vi "Main - Auto Detect Modules.vi"(8 "error in (no error)":errorcluster, 11 "Node Ptr":u64 format="%.0x") -> (0 "error out":errorcluster)   [LabVIEW 2016, in "Scan Engine Custom Device.lvlib"]
uses:
  Scan Engine Custom Device.lvlib
  <vilib>/NI Veristand/Custom Device API/Custom Device Channel.ctl
  <vilib>/NI Veristand/Custom Device API/Custom Device Channel Type.ctl
  Modules.lvlibp/RSI Module/Slot Settings.ctl
  Modules.lvlibp/RSI Module/Module Models.ctl
  Type Defs/Host - FPGAScanInterfaceMode.ctl
  Globals/String Constants.vi
  Globals/Scan Engine GUIDs.vi
  Globals/Property Strings.vi
  Modules.lvlibp/RSI Module/Class Property Strings.vi
  Modules.lvlibp/RSI Module/RSI Module.lvclass
  Modules.lvlibp/RemIO Module/RemIO Module.lvclass
  <vilib>/NI Veristand/Custom Device API/Custom Device API.lvlib
  Modules.lvlibp
  <resource>/objmgr/ni.var.rc
panel:
  in  "Tag":string
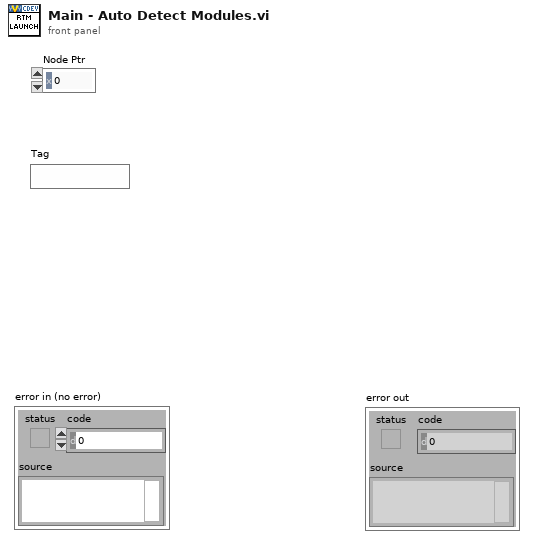
[diagram p1: front panel]
types:
  T1 = typedef "Custom Device API.lvlib/Custom Device Channel Type.ctl" = enum16{"Input", "Output"}
  T2 = typedef "Modules.lvlibp/RSI Module.lvclass/Slot Settings.ctl" = cluster{"Slot":u32, "EtherCAT?":bool}
  T3 = typedef "Modules.lvlibp/RSI Module.lvclass/Module Models.ctl" = enum16{"Empty", "NI 9201", "NI 9203", "NI 9205", "NI 9206", "NI 9207", "NI 9208", "NI 9211", "NI 9212", "NI 9213", "NI 9214", "NI 9215", "NI 9217", "NI 9219", "NI 9220", "NI 9221", "NI 9222", "NI 9223", "NI 9225", "NI 9227", "NI 9229", "NI 9233", "NI 9234", "NI 9235", "NI 9236", "NI 9237", "NI 9239", "NI 9242", "NI 9244", "NI 9263", "NI 9264", "NI 9265", "NI 9269", "NI 9375", "NI 9401", "NI 9402", "NI 9403", "NI 9411", "NI 9421", "NI 9422", "NI 9423", "NI 9425", "NI 9426", "NI 9435", "NI 9437", "NI 9472", "NI 9474", "NI 9475", "NI 9476", "NI 9477", "NI 9478", "NI 9481", "NI 9482", "NI 9485"}
  T4 = typedef "Scan Engine Custom Device.lvlib/Host - FPGAScanInterfaceMode.ctl" = enum16{"Use Current", "FPGA", "Scan Mode"}
  T5 = typedef "Custom Device API.lvlib/Custom Device Item Ref.ctl" = u64
  T6 = typedef "Custom Device API.lvlib/Custom Device Item Info.ctl" = cluster{"Name":string, "Is Channel":bool, "GUID":string, "Is Waveform":bool}
  T7 = typedef "Scan Engine Custom Device.lvlib/Host - HW Config.ctl" = cluster{"Local Chassis":T8, "Masters":T10[]}
  T8 = typedef "Scan Engine Custom Device.lvlib/Host - Local Chassis.ctl" = cluster{"Modules":T9[]}
  T9 = typedef "Scan Engine Custom Device.lvlib/Host - Module.ctl" = cluster{"IOV Ref":refnum<k21>, "Slot":u32, "Model":u32}
  T10 = typedef "Scan Engine Custom Device.lvlib/Host - Master.ctl" = cluster{"IOV Ref":refnum<k21>, "Name":string, "Master ID":u32, "Slaves":T11[]}
  T11 = typedef "Scan Engine Custom Device.lvlib/Host - Slave.ctl" = cluster{"IOV Ref":refnum<k21>, "Name":string, "Position Address":u16, "Bitfile Signature":u8[], "Modules":T9[], "ECAT Variablenobjekt":refnum<k21>[]}
  T12 = typedef "Custom Device API.lvlib/Custom Device Channel.ctl" = cluster{"Type":T1, "Units":string, "Default Value":dbl, "Faultable":bool, "Scalable":bool}
  T13 = typedef "Scan Engine Custom Device.lvlib/ECAT Channel Data Type.ctl" = enum16{"Boolean", "Fixed Point", "Int8", "Int16", "Int32", "Int64", "U32 Bit Field", "UInt8", "UInt16", "UInt32", "UInt64", "Other", "DBL"}
  T14 = typedef "Modules.lvlibp/Custom Device API.lvlib/Custom Device Item Ref.ctl" = u64
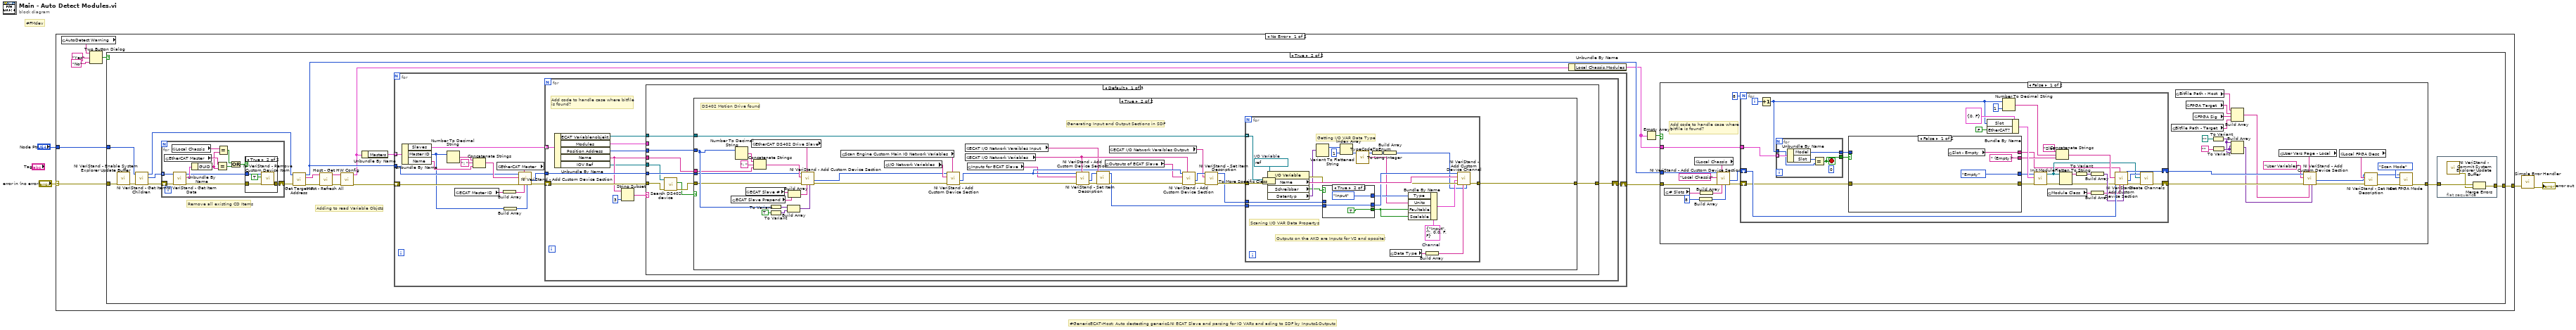
[diagram p0: block diagram]
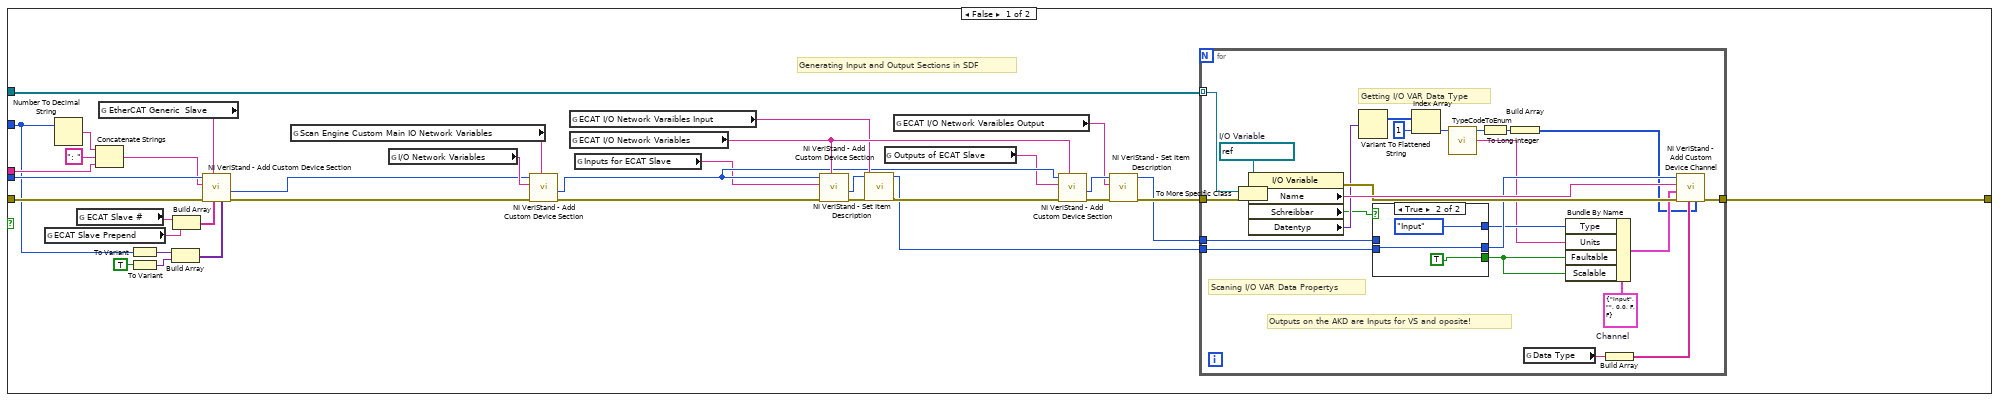
[diagram p3: hidden frame]
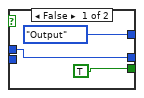
[diagram p4: hidden frame]
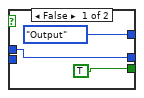
[diagram p5: hidden frame]
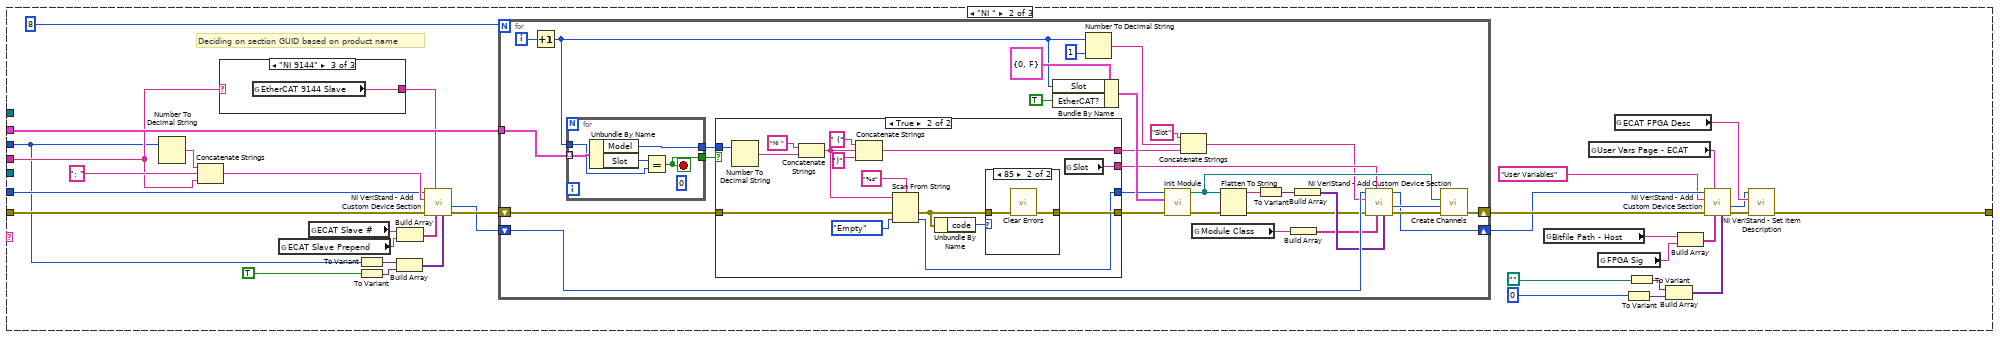
[diagram p6: hidden frame]
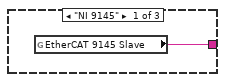
[diagram p7: hidden frame]
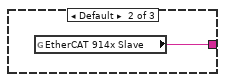
[diagram p8: hidden frame]
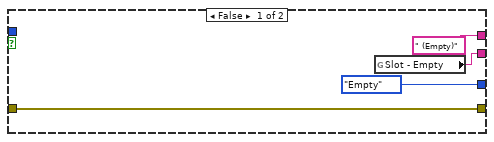
[diagram p9: hidden frame]
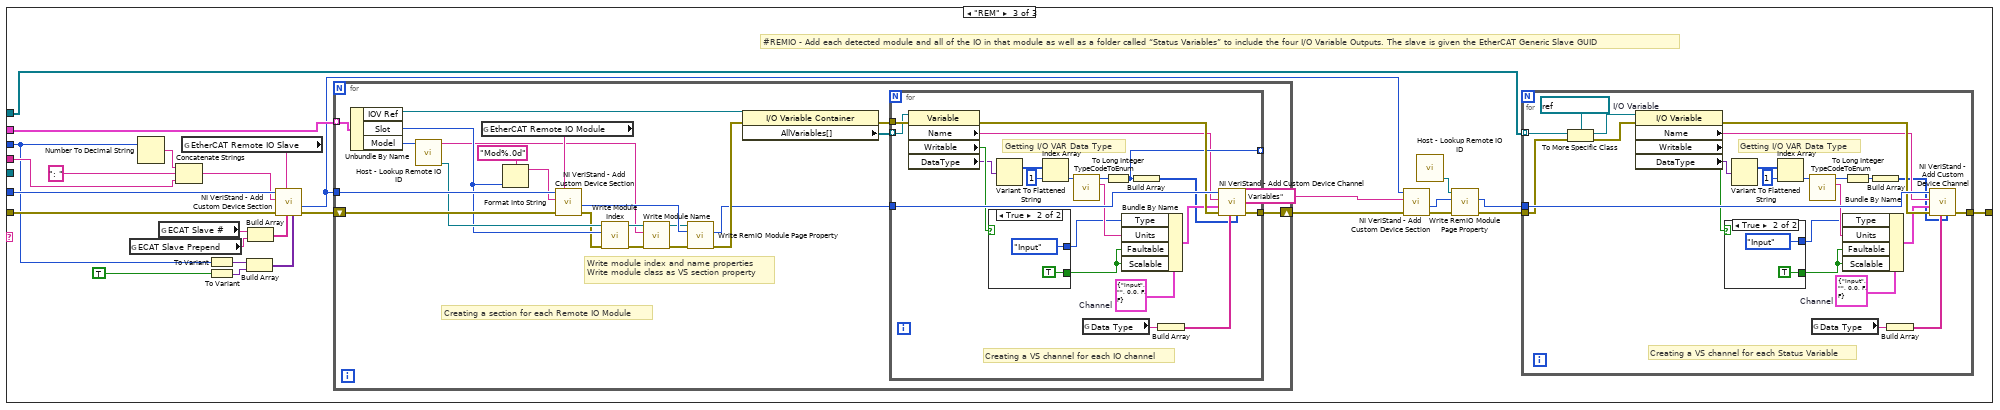
[diagram p11: hidden frame]
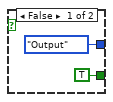
[diagram p12: hidden frame]
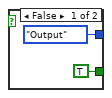
[diagram p13: hidden frame]
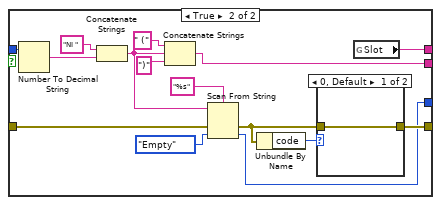
[diagram p15: hidden frame]
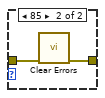
[diagram p16: hidden frame]
diagram:
  # "#FMdev"
  # "#GenericECAT-Host: Auto dectecting generic&NI ECAT Slave and parsing for IO VARs and ading to SDF by Inputs&Outputs"
  n1 = case shown="No Error" "error in (no error)" {
    selector: "error in (no error)" -> [w6 w512]
    tunnel: "Node Ptr" -> [w7 _]
    tunnel: [w5 w512] -> w2
    frame No Error {
      n2 = global read "String Constants.vi" "AutoDetect Warning"() -> (w8:string)
      n3 = Two Button Dialog(message=w8, 1:"No" ("F button name (\"Cancel\")"), 2:"Yes" ("T button name (\"OK\")")) -> (T button?=w11:bool)
      n4 = case shown="True" w11 {
        tunnel: w6 -> [w12 w26]
        tunnel: [w12 w14] -> w5
        tunnel: w7 -> [_ w30]
        frame False {
        }
        frame True {
          # "Adding to read Variable Objcts"
          # "Remove all existing CD Items"
          n5 = call <vilib>:"NI VeriStand - Enable System Explorer Update Buffer.vi"("error in (no error)"=w26) -> ("error out"=w25:errorcluster)  [unwired: 10 in]
          n6 = call <vilib>:"NI VeriStand - Get Item Children.vi"("error in (no error)"=w25, "Item Ref in"=w30) -> ("error out"=w31:errorcluster, "Child Refs"=w32:T5[], "Item Ref out"=w29:T5)  [unwired: 6 in, 1 out]
          n7 = for {
            tunnel: w32 -> [w415] mode=indexing
            shift-right: [w409] -> w13
            shift-left: w31 -> [w414]
            n8 = global read "Scan Engine GUIDs.vi" "EtherCAT Master"() -> (w412:string)
            n9 = global read "Scan Engine GUIDs.vi" "Local Chassis"() -> (w408:string)
            n10 = call <vilib>:"NI VeriStand - Get Item Data.vi"("error in (no error)"=w414, "Item Ref in"=w415) -> ("error out"=w410:errorcluster, "Item Info"=w413:T6, "Item Ref out"=w411:T5)  [unwired: 6 in, 1 out]
            n11 = Unbundle By Name(w413) -> ("GUID"=w407:string)
            n12 = Equal?(x=w412, y=w407) -> (x = y?=w405:bool)
            n13 = Equal?(x=w408, y=w407) -> (x = y?=w406:bool)
            n14 = Or(x=w406, y=w405) -> (x .or. y?=w404:bool)
            n15 = case shown="True" w404 {
              tunnel: w411 -> [_ w419]
              tunnel: w410 -> [w416 w420]
              tunnel: [w416 w418] -> w409
              frame False {
              }
              frame True {
                n16 = call <vilib>:"NI VeriStand - Remove Custom Device Item.vi"("error in (no error)"=w420, "Force Delete (F)"=TRUE, "Item Ref in"=w419) -> ("error out"=w418:errorcluster)  [unwired: 7 in, 1 out]
              }
            }
          }
          n17 = call "Get Target IP Address.vi"("error in"=w13, "Item Ref in"=w29) -> ("error out"=w27:errorcluster, "Target IP Address"=w28:string, "Item Ref out"=w19:T5)  [unwired: 7 in]
          n18 = call "Host - Refresh All.vi"("error in (no error)"=w27, "serverName"=w28) -> ("error out"=w24:errorcluster, "serverName"=w22:string)  [unwired: 8 in]
          n19 = call "Host - Get HW Config.vi"("error in (no error)"=w24, "serverName"=w22) -> ("error out"=w23:errorcluster, "HW Config"=w18:T7)  [unwired: 8 in]
          n20 = Unbundle By Name(w18) -> ("Masters"=w21:T10[])
          n21 = for {
            tunnel: w21 -> [w46] mode=indexing
            shift-right: [w36] -> w20
            shift-left: w23 -> [w47]
            tunnel: w19 -> [w48]
            n22 = Unbundle By Name(w46) -> ("Slaves"=w38:T11[], "Master ID"=w41:u32, "Name"=w43:string)
            n23 = Number To Decimal String(number=w41) -> (decimal integer string=w45:string)  [unwired: 1 in]
            n24 = global read "Property Strings.vi" "ECAT Master ID"() -> (w42:string)
            n25 = Concatenate Strings(w45, ": " ("string"), w43) -> (w49:string)
            n26 = global read "Scan Engine GUIDs.vi" "EtherCAT Master"() -> (w51:string)
            n27 = Build Array(w42) -> (w50:string[])
            n28 = Build Array(w41) -> (w40:u32[])
            n29 = call <vilib>:"NI VeriStand - Add Custom Device Section.vi"("Property Values"=w40, "Property names"=w50, "GUID (Default Section)"=w51, "error in (no error)"=w47, "Section Name"=w49, "Parent Ref in"=w48) -> ("error out"=w39:errorcluster, "Section Ptr"=w37:T5)  [unwired: 2 in, 2 out]
            n30 = for {
              shift-right: [w58] -> w36
              shift-left: w39 -> [w61]
              tunnel: w38 -> [w62] mode=indexing
              tunnel: w37 -> [w60]
              # "Add code to handle case where bitfile\nis found?"
              n31 = Unbundle By Name(w62) -> ("ECAT Variablenobjekt"=w56:refnum<k21>[], "Modules"=w59:T9[], "Position Address"=w54:u16, "Name"=w53:string, "IOV Ref"=w52:refnum<k21>)
              n32 = String Subset(string=w53, length (rest)=3 ("Länge (Rest)")) -> (substring=w55:string)  [unwired: 1 in]
              n33 = case shown="Default" w55 {
                tunnel: w61 -> [w66 w226 w318]
                tunnel: w59 -> [_ w225 w328]
                tunnel: [w70 w224 w325] -> w58
                tunnel: w56 -> [w71 _ w324]
                tunnel: w60 -> [w69 w211 w315]
                tunnel: w54 -> [w67 w208 w302]
                tunnel: w53 -> [w68 w210 w305]
                tunnel: w52 -> [w65 _ _]
                frame Default {
                  n34 = call "Search DS402 device.vi"("error in (no error)"=w66, "Slave Reference In"=w65) -> ("error out"=w64:errorcluster, "Found"=w63:bool)  [unwired: 7 in, 1 out]
                  n35 = case shown="True" w63 {
                    tunnel: w71 -> [w107 w144]
                    tunnel: [w106 w142] -> w70
                    tunnel: w64 -> [w89 w143]
                    tunnel: w69 -> [w88 w140]
                    tunnel: w68 -> [w75 w141]
                    tunnel: w67 -> [w72 w145]
                    frame False {
                      # "Generating Input and Output Sections in SDF"
                      n36 = global read "Property Strings.vi" "ECAT Slave Prepend"() -> (w79:string)
                      n37 = Number To Decimal String(number=w72) -> (decimal integer string=w82:string)  [unwired: 1 in]
                      n38 = global read "Property Strings.vi" "ECAT Slave #"() -> (w80:string)
                      n39 = Concatenate Strings(w82, ": " ("string"), w75) -> (w84:string)
                      n40 = global read "Scan Engine GUIDs.vi" "EtherCAT Generic  Slave"() -> (w85:string)
                      n41 = To Variant(anything=w72) -> (Variant=w78:variant)
                      n42 = To Variant(anything=TRUE) -> (Variant=w77:variant)
                      n43 = Build Array(w78, w77) -> (w74:variant[])
                      n44 = Build Array(w80, w79) -> (w81:string[])
                      n45 = call <vilib>:"NI VeriStand - Add Custom Device Section.vi"("Property Values"=w74, "Property names"=w81, "GUID (Default Section)"=w85, "error in (no error)"=w89, "Section Name"=w84, "Parent Ref in"=w88) -> ("error out"=w86:errorcluster, "Section Ptr"=w87:T5)  [unwired: 2 in, 2 out]
                      n46 = global read "Scan Engine GUIDs.vi" "Scan Engine Custom Main IO Network Variables"() -> (w99:string)
                      n47 = global read "Property Strings.vi" "I/O Network Variables"() -> (w92:string)
                      n48 = call <vilib>:"NI VeriStand - Add Custom Device Section.vi"("GUID (Default Section)"=w99, "error in (no error)"=w86, "Section Name"=w92, "Parent Ref in"=w87) -> ("error out"=w93:errorcluster, "Section Ptr"=w94:T5)  [unwired: 4 in, 2 out]
                      n49 = global read "String Constants.vi" "ECAT I/O Network Varaibles Input"() -> (w95:string)
                      n50 = global read "Scan Engine GUIDs.vi" "ECAT I/O Network Variables"() -> (w96:string)
                      n51 = global read "Property Strings.vi" "Inputs for ECAT Slave"() -> (w91:string)
                      n52 = call <vilib>:"NI VeriStand - Add Custom Device Section.vi"("GUID (Default Section)"=w96, "error in (no error)"=w93, "Section Name"=w91, "Parent Ref in"=w94) -> ("error out"=w105:errorcluster, "Section Ptr"=w98:T5)  [unwired: 4 in, 2 out]
                      n53 = call <vilib>:"NI VeriStand - Set Item Description.vi"("error in (no error)"=w105, "Description"=w95, "Item Ref in"=w98) -> ("error out"=w104:errorcluster, "Item Ref out"=w103:T5)  [unwired: 6 in, 1 out]
                      n54 = global read "Property Strings.vi" "Outputs of ECAT Slave"() -> (w90:string)
                      n55 = global read "String Constants.vi" "ECAT I/O Network Varaibles Output"() -> (w73:string)
                      n56 = call <vilib>:"NI VeriStand - Add Custom Device Section.vi"("GUID (Default Section)"=w96, "error in (no error)"=w104, "Section Name"=w90, "Parent Ref in"=w94) -> ("error out"=w102:errorcluster, "Section Ptr"=w97:T5)  [unwired: 4 in, 2 out]
                      n57 = call <vilib>:"NI VeriStand - Set Item Description.vi"("error in (no error)"=w102, "Description"=w73, "Item Ref in"=w97) -> ("error out"=w101:errorcluster, "Item Ref out"=w100:T5)  [unwired: 6 in, 1 out]
                      n58 = for {
                        tunnel: w107 -> [w127] mode=indexing
                        tunnel: [w131] -> w106
                        tunnel: w101 -> [w120]
                        tunnel: w100 -> [w118]
                        tunnel: w103 -> [w116]
                        w126 = refnum<k21> refnum  # I/O Variable
                        w130 = T12 {"Type"=enum."Input", "Units"="", "Default Value"=0.0, "Faultable"=FALSE, "Scalable"=FALSE}  # Channel
                        # "Getting I/O VAR Data Type"
                        # "Scaning I/O VAR Data Propertys"
                        # "Outputs on the AKD are Inputs for VS and oposite!"
                        n59 = To More Specific Class(target class=w126, reference=w127, error in=w120) -> (specific class reference=w125:refnum<k21>, error out=w124:errorcluster)
                        n60 = property class="I/O Variable"(reference=w125, error in=w124) -> (error out=w132:errorcluster, "Name"=w133:string, "Schreibbar"=w119:bool, "Datentyp"=w123:variant)  [unwired: 1 out]
                        n61 = Variant To Flattened String(Variant=w123) -> (1:w122:i16[])  [unwired: 1 out]
                        n62 = case shown="True" w119 {
                          tunnel: [Custom_Device_Channel_Type."Output" ("Type") Custom_Device_Channel_Type."Input" ("Type")] -> w112
                          tunnel: [w134 w137] -> w117
                          tunnel: w118 -> [w134 _]
                          tunnel: w116 -> [_ w137]
                          tunnel: [TRUE TRUE] -> w115
                          frame False {
                          }
                          frame True {
                          }
                        }
                        n63 = Index Array(array=w122, index=1) -> (element=w110:i16)
                        n64 = call "TypeCodeToEnum.vi"("Type Code (numbers in hexadecimal)"=w110) -> (2:"UDV Data Type"=w111:string, 3:"UDV Data Type"=w108:T13)  [unwired: 9 in]
                        n65 = To Long Integer(number=w108) -> (32bit integer=w109:i32)
                        n66 = Build Array(w109) -> (w113:i32[])
                        n67 = global read "Property Strings.vi" "Data Type"() -> (w114:string)
                        n68 = Bundle By Name(cluster=w130, "Type"=w112, "Units"=w111, "Faultable"=w115, "Scalable"=w115) -> (w129:T12)
                        n69 = Build Array(w114) -> (w128:string[])
                        n70 = call <vilib>:"NI VeriStand - Add Custom Device Channel.vi"("Property Values"=w113, "Property names"=w128, "error in (no error)"=w132, "Channel"=w129, "Channel Name"=w133, "Parent Ref in"=w117) -> ("error out"=w131:errorcluster)  [unwired: 2 in, 3 out]
                      }
                    }
                    frame True {
                      # "Generating Input and Output Sections in SDF"
                      # "DS402 Motion Drive found"
                      n71 = global read "Property Strings.vi" "ECAT Slave Prepend"() -> (w151:string)
                      n72 = Number To Decimal String(number=w145) -> (decimal integer string=w154:string)  [unwired: 1 in]
                      n73 = global read "Property Strings.vi" "ECAT Slave #"() -> (w152:string)
                      n74 = global read "Scan Engine GUIDs.vi" "EtherCAT DS402 Drive Slave"() -> (w157:string)
                      n75 = Concatenate Strings(w154, ": " ("string"), w141) -> (w156:string)
                      n76 = To Variant(anything=w145) -> (Variant=w150:variant)
                      n77 = To Variant(anything=TRUE) -> (Variant=w149:variant)
                      n78 = Build Array(w150, w149) -> (w147:variant[])
                      n79 = Build Array(w152, w151) -> (w153:string[])
                      n80 = call <vilib>:"NI VeriStand - Add Custom Device Section.vi"("Property Values"=w147, "Property names"=w153, "GUID (Default Section)"=w157, "error in (no error)"=w143, "Section Name"=w156, "Parent Ref in"=w140) -> ("error out"=w158:errorcluster, "Section Ptr"=w159:T5)  [unwired: 2 in, 2 out]
                      n81 = global read "Scan Engine GUIDs.vi" "Scan Engine Custom Main IO Network Variables"() -> (w169:string)
                      n82 = global read "Property Strings.vi" "I/O Network Variables"() -> (w162:string)
                      n83 = call <vilib>:"NI VeriStand - Add Custom Device Section.vi"("GUID (Default Section)"=w169, "error in (no error)"=w158, "Section Name"=w162, "Parent Ref in"=w159) -> ("error out"=w163:errorcluster, "Section Ptr"=w164:T5)  [unwired: 4 in, 2 out]
                      n84 = global read "String Constants.vi" "ECAT I/O Network Varaibles Input"() -> (w165:string)
                      n85 = global read "Scan Engine GUIDs.vi" "ECAT I/O Network Variables"() -> (w166:string)
                      n86 = global read "Property Strings.vi" "Inputs for ECAT Slave"() -> (w161:string)
                      n87 = call <vilib>:"NI VeriStand - Add Custom Device Section.vi"("GUID (Default Section)"=w166, "error in (no error)"=w163, "Section Name"=w161, "Parent Ref in"=w164) -> ("error out"=w175:errorcluster, "Section Ptr"=w168:T5)  [unwired: 4 in, 2 out]
                      n88 = call <vilib>:"NI VeriStand - Set Item Description.vi"("error in (no error)"=w175, "Description"=w165, "Item Ref in"=w168) -> ("error out"=w174:errorcluster, "Item Ref out"=w173:T5)  [unwired: 6 in, 1 out]
                      n89 = global read "Property Strings.vi" "Outputs of ECAT Slave"() -> (w160:string)
                      n90 = global read "String Constants.vi" "ECAT I/O Network Varaibles Output"() -> (w146:string)
                      n91 = call <vilib>:"NI VeriStand - Add Custom Device Section.vi"("GUID (Default Section)"=w166, "error in (no error)"=w174, "Section Name"=w160, "Parent Ref in"=w164) -> ("error out"=w172:errorcluster, "Section Ptr"=w167:T5)  [unwired: 4 in, 2 out]
                      n92 = call <vilib>:"NI VeriStand - Set Item Description.vi"("error in (no error)"=w172, "Description"=w146, "Item Ref in"=w167) -> ("error out"=w171:errorcluster, "Item Ref out"=w170:T5)  [unwired: 6 in, 1 out]
                      n93 = for {
                        tunnel: w144 -> [w195] mode=indexing
                        tunnel: [w199] -> w142
                        tunnel: w171 -> [w188]
                        tunnel: w170 -> [w186]
                        tunnel: w173 -> [w184]
                        w194 = refnum<k21> refnum  # I/O Variable
                        w198 = T12 {"Type"=enum."Input", "Units"="", "Default Value"=0.0, "Faultable"=FALSE, "Scalable"=FALSE}  # Channel
                        # "Getting I/O VAR Data Type"
                        # "Scaning I/O VAR Data Propertys"
                        # "Outputs on the AKD are Inputs for VS and oposite!"
                        n94 = To More Specific Class(target class=w194, reference=w195, error in=w188) -> (specific class reference=w193:refnum<k21>, error out=w192:errorcluster)
                        n95 = property class="I/O Variable"(reference=w193, error in=w192) -> (error out=w200:errorcluster, "Name"=w201:string, "Schreibbar"=w187:bool, "Datentyp"=w191:variant)  [unwired: 1 out]
                        n96 = Variant To Flattened String(Variant=w191) -> (1:w190:i16[])  [unwired: 1 out]
                        n97 = case shown="True" w187 {
                          tunnel: [Custom_Device_Channel_Type."Output" ("Type") Custom_Device_Channel_Type."Input" ("Type")] -> w180
                          tunnel: [w202 w205] -> w185
                          tunnel: w186 -> [w202 _]
                          tunnel: w184 -> [_ w205]
                          tunnel: [TRUE TRUE] -> w183
                          frame False {
                          }
                          frame True {
                          }
                        }
                        n98 = Index Array(array=w190, index=1) -> (element=w178:i16)
                        n99 = call "TypeCodeToEnum.vi"("Type Code (numbers in hexadecimal)"=w178) -> (2:"UDV Data Type"=w179:string, 3:"UDV Data Type"=w176:T13)  [unwired: 9 in]
                        n100 = To Long Integer(number=w176) -> (32bit integer=w177:i32)
                        n101 = Build Array(w177) -> (w181:i32[])
                        n102 = global read "Property Strings.vi" "Data Type"() -> (w182:string)
                        n103 = Bundle By Name(cluster=w198, "Type"=w180, "Units"=w179, "Faultable"=w183, "Scalable"=w183) -> (w197:T12)
                        n104 = Build Array(w182) -> (w196:string[])
                        n105 = call <vilib>:"NI VeriStand - Add Custom Device Channel.vi"("Property Values"=w181, "Property names"=w196, "error in (no error)"=w200, "Channel"=w197, "Channel Name"=w201, "Parent Ref in"=w185) -> ("error out"=w199:errorcluster)  [unwired: 2 in, 3 out]
                      }
                    }
                  }
                }
                frame "NI " {
                  # "Deciding on section GUID based on product name"
                  n106 = Number To Decimal String(number=w208) -> (decimal integer string=w222:string)  [unwired: 1 in]
                  n107 = Concatenate Strings(w222, ": " ("string"), w210) -> (w220:string)
                  n108 = case shown="\"NI 9144\"" w210 {
                    tunnel: [w242 w243 w244] -> w209
                    frame "NI 9145" {
                      n109 = global read "Scan Engine GUIDs.vi" "EtherCAT 9145 Slave"() -> (w242:string)
                    }
                    frame Default {
                      n110 = global read "Scan Engine GUIDs.vi" "EtherCAT 914x Slave"() -> (w243:string)
                    }
                    frame "NI 9144" {
                      n111 = global read "Scan Engine GUIDs.vi" "EtherCAT 9144 Slave"() -> (w244:string)
                    }
                  }
                  n112 = global read "Property Strings.vi" "ECAT Slave Prepend"() -> (w218:string)
                  n113 = global read "Property Strings.vi" "ECAT Slave #"() -> (w217:string)
                  n114 = To Variant(anything=w208) -> (Variant=w219:variant)
                  n115 = To Variant(anything=TRUE) -> (Variant=w213:variant)
                  n116 = Build Array(w219, w213) -> (w215:variant[])
                  n117 = Build Array(w217, w218) -> (w216:string[])
                  n118 = call <vilib>:"NI VeriStand - Add Custom Device Section.vi"("Property Values"=w215, "Property names"=w216, "GUID (Default Section)"=w209, "Section Name"=w220, "Parent Ref in"=w211) -> ("Section Ptr"=w212:T5)  [unwired: 3 in, 3 out]
                  n119 = for {
                    N: 8 -> [_]
                    shift-right: [w248] -> w237
                    shift-left: w226 -> [w254]
                    shift-right: [w246] -> w236
                    shift-left: w212 -> [w274]
                    tunnel: w225 -> [w259]
                    i -> [w271]
                    n120 = Increment(x=w271) -> (x+1=w258:i32)
                    n121 = for {
                      tunnel: w259 -> [w301] mode=indexing
                      tunnel: w258 -> [w299]
                      tunnel: [w298] -> w257
                      tunnel: [w297] -> w252
                      stop <- w298 stop-if-true
                      (unwired) u32 0 ("Model")
                      n122 = Unbundle By Name(w301) -> ("Model"=w297:u32, "Slot"=w300:u32)
                      n123 = Equal?(x=w300, y=w299) -> (x = y?=w298:bool)
                    }
                    n124 = case shown="True" w257 {
                      tunnel: [" (Empty)" ("Section Name") w280] -> w256
                      tunnel: [Module_Models."Empty" ("Module") w287] -> w255
                      tunnel: w254 -> [w276 w288]
                      tunnel: [w276 w289] -> w253
                      tunnel: w252 -> [_ w286]
                      tunnel: [w275 w279] -> w247
                      frame False {
                        n125 = global read "Scan Engine GUIDs.vi" "Slot - Empty"() -> (w275:string)
                      }
                      frame True {
                        n126 = Number To Decimal String(number=w286) -> (decimal integer string=w285:string)  [unwired: 1 in]
                        n127 = Concatenate Strings("NI " ("string"), w285) -> (w283:string)
                        n128 = Concatenate Strings(" (" ("string"), w283, ")" ("string")) -> (w280:string)
                        n129 = Scan From String(format string="%s", input string=w283, error in=w288, default 1=Module_Models."Empty" ("Module")) -> (error out=w290:errorcluster, output 1=w287:T3)  [unwired: 1 in, 2 out]
                        n130 = Unbundle By Name(w290) -> ("code"=w291:i32)
                        n131 = case shown="85" w291 {
                          tunnel: [w294 w295] -> w289
                          tunnel: w290 -> [w294 w296]
                          frame 0, Default {
                          }
                          frame 85 {
                            n132 = call <vilib>:"Clear Errors.vi"("error in (no error)"=w296) -> ("error out"=w295:errorcluster)  [unwired: 5 in, 1 out]
                          }
                        }
                        n133 = global read "Scan Engine GUIDs.vi" "Slot"() -> (w279:string)
                      }
                    }
                    n134 = Bundle By Name(cluster=T2 {"Slot"=0, "EtherCAT?"=FALSE} ("Slot Settings"), "Slot"=w258, "EtherCAT?"=TRUE) -> (w268:T2)
                    n135 = Number To Decimal String(number=w258, width (-)=i16 1) -> (decimal integer string=w273:string)
                    n136 = call "Init Module.vi"("error in (no error)"=w253, "Slot Settings"=w268, "Module Model"=w255) -> ("error out"=w263:errorcluster, "RSI Module out"=w249:refnum<class "RSI Module.lvclass">)  [unwired: 7 in]
                    n137 = Concatenate Strings("Slot" ("string"), w273, w256) -> (w245:string)
                    n138 = global read "Class Property Strings.vi" "Module Class"() -> (w261:string)
                    n139 = Flatten To String(anything=w249, error in (no error)=w263) -> (data string=w264:string, error out=w262:errorcluster)  [unwired: 2 in, 1 out]
                    n140 = To Variant(anything=w264) -> (Variant=w269:variant)
                    n141 = Build Array(w261) -> (w265:string[])
                    n142 = Build Array(w269) -> (w270:variant[])
                    n143 = call <vilib>:"NI VeriStand - Add Custom Device Section.vi"("Property Values"=w270, "Property names"=w265, "GUID (Default Section)"=w247, "error in (no error)"=w262, "Section Name"=w245, "Parent Ref in"=w274) -> ("error out"=w250:errorcluster, "Section Ptr"=w251:T5, "Parent Ref out"=w246:T5)  [unwired: 2 in, 1 out]
                    n144 = call-dynamic "Create Channels.vi"("error in (no error)"=w250, "RSI Module in"=w249, "Parent Ref in"=w251) -> ("error out"=w248:errorcluster)  [unwired: 6 in, 2 out]
                  }
                  n145 = global read "Property Strings.vi" "Bitfile Path - Host"() -> (w228:string)
                  n146 = global read "Scan Engine GUIDs.vi" "User Vars Page - ECAT"() -> (w239:string)
                  n147 = global read "Property Strings.vi" "FPGA Sig"() -> (w227:string)
                  n148 = global read "String Constants.vi" "ECAT FPGA Desc"() -> (w238:string)
                  n149 = To Variant(anything=u32 0 ("ModuleIdent (ECAT)")) -> (Variant=w229:variant)
                  n150 = To Variant(anything=path "") -> (Variant=w230:variant)
                  n151 = Build Array(w230, w229) -> (w240:variant[])
                  n152 = Build Array(w228, w227) -> (w241:string[])
                  n153 = call <vilib>:"NI VeriStand - Add Custom Device Section.vi"("Property Values"=w240, "Property names"=w241, "GUID (Default Section)"=w239, "error in (no error)"=w237, "Section Name"="User Variables", "Parent Ref in"=w236) -> ("error out"=w233:errorcluster, "Section Ptr"=w234:T5)  [unwired: 2 in, 2 out]
                  n154 = call <vilib>:"NI VeriStand - Set Item Description.vi"("error in (no error)"=w233, "Description"=w238, "Item Ref in"=w234) -> ("error out"=w224:errorcluster)  [unwired: 6 in, 2 out]
                }
                frame "REM" {
                  # "#REMIO - Add each detected module and all of the IO in that module as well as a folder called “Status Variables” to include the four I/O Variable Outputs. The slave is given the EtherCAT Generic Slave GUID"
                  n155 = global read "Property Strings.vi" "ECAT Slave Prepend"() -> (w309:string)
                  n156 = Number To Decimal String(number=w302) -> (decimal integer string=w313:string)  [unwired: 1 in]
                  n157 = global read "Property Strings.vi" "ECAT Slave #"() -> (w308:string)
                  n158 = Concatenate Strings(w313, ": " ("string"), w305) -> (w311:string)
                  n159 = global read "Scan Engine GUIDs.vi" "EtherCAT Remote IO Slave"() -> (w314:string)
                  n160 = To Variant(anything=w302) -> (Variant=w310:variant)
                  n161 = To Variant(anything=TRUE) -> (Variant=w303:variant)
                  n162 = Build Array(w310, w303) -> (w306:variant[])
                  n163 = Build Array(w308, w309) -> (w307:string[])
                  n164 = call <vilib>:"NI VeriStand - Add Custom Device Section.vi"("Property Values"=w306, "Property names"=w307, "GUID (Default Section)"=w314, "error in (no error)"=w318, "Section Name"=w311, "Parent Ref in"=w315) -> ("error out"=w317:errorcluster, "Section Ptr"=w316:T5)  [unwired: 2 in, 2 out]
                  n165 = for {
                    shift-right: [w344] -> w327
                    shift-left: w317 -> [w350]
                    tunnel: w316 -> [w349]
                    tunnel: w328 -> [w348] mode=indexing
                    # "Write module index and name properties\nWrite module class as VS section property"
                    # "Creating a section for each Remote IO Module"
                    n166 = Unbundle By Name(w348) -> ("IOV Ref"=w347:refnum<k21>, "Slot"=w340:u32, "Model"=w343:u32)
                    n167 = call "Host - Lookup Remote IO ID.vi"("Module ID"=w343) -> ("RemIO Module Out"=w341:refnum<class "RemIO Module.lvclass">, "Module Name"=w329:string)  [unwired: 9 in]
                    n168 = global read "Scan Engine GUIDs.vi" "EtherCAT Remote IO Module"() -> (w339:string)
                    n169 = Format Into String(format string="Mod%.0d", w340) -> (resulting string=w335:string)  [unwired: 2 in, 1 out]
                    n170 = call <vilib>:"NI VeriStand - Add Custom Device Section.vi"("GUID (Default Section)"=w339, "error in (no error)"=w350, "Section Name"=w335, "Parent Ref in"=w349) -> ("error out"=w337:errorcluster, "Section Ptr"=w338:T5)  [unwired: 4 in, 2 out]
                    n171 = call-dynamic "Write Module Index.vi"("error in (no error)"=w337, "Module Index"=w340, "RemIO Module in"=w341) -> ("error out"=w332:errorcluster, "RemIO Module out"=w333:refnum<class "RemIO Module.lvclass">)  [unwired: 7 in]
                    n172 = call-dynamic "Write Module Name.vi"("error in (no error)"=w332, "Module Name"=w329, "RemIO Module in"=w333) -> ("error out"=w331:errorcluster, "RemIO Module out"=w330:refnum<class "RemIO Module.lvclass">)  [unwired: 7 in]
                    n173 = call "Write RemIO Module Page Property.vi"("error in (no error)"=w331, "Node Ptr In"=w338, "RemIO Module"=w330) -> ("error out"=w342:errorcluster, "Node Ptr Out"=w336:T14)  [unwired: 6 in, 1 out]
                    n174 = property class="I/O Variable Container"(reference=w347, error in=w342) -> (error out=w345:errorcluster, "AllVariables[]"=w346:refnum<k21>[])  [unwired: 1 out]
                    n175 = for {
                      tunnel: w346 -> [w369] mode=indexing
                      tunnel: w336 -> [w371]
                      tunnel: w345 -> [w370]
                      tunnel: [w353] -> w344
                      tunnel: [w352] -> _ mode=indexing
                      w367 = T12 {"Type"=enum."Input", "Units"="", "Default Value"=0.0, "Faultable"=FALSE, "Scalable"=FALSE}  # Channel
                      # "Creating a VS channel for each IO channel"
                      # "Getting I/O VAR Data Type"
                      n176 = property class="Variable"(reference=w369, error in=w370) -> (error out=w368:errorcluster, "Name"=w351:string, "Writable"=w366:bool, "DataType"=w361:variant)  [unwired: 1 out]
                      n177 = case shown="True" w366 {
                        tunnel: [TRUE TRUE] -> w365
                        tunnel: [Custom_Device_Channel_Type."Output" ("Type") Custom_Device_Channel_Type."Input" ("Type")] -> w354
                        frame False {
                        }
                        frame True {
                        }
                      }
                      n178 = Variant To Flattened String(Variant=w361) -> (1:w362:i16[])  [unwired: 1 out]
                      n179 = Index Array(array=w362, index=1) -> (element=w364:i16)
                      n180 = call "TypeCodeToEnum.vi"("Type Code (numbers in hexadecimal)"=w364) -> (2:"UDV Data Type"=w360:string, 3:"UDV Data Type"=w358:T13)  [unwired: 9 in]
                      n181 = global read "Property Strings.vi" "Data Type"() -> (w357:string)
                      n182 = To Long Integer(number=w358) -> (32bit integer=w352:i32)
                      n183 = Bundle By Name(cluster=w367, "Type"=w354, "Units"=w360, "Faultable"=w365, "Scalable"=w365) -> (w359:T12)
                      n184 = Build Array(w352) -> (w355:i32[])
                      n185 = Build Array(w357) -> (w356:string[])
                      n186 = call <vilib>:"NI VeriStand - Add Custom Device Channel.vi"("Property Values"=w355, "Property names"=w356, "error in (no error)"=w368, "Channel"=w359, "Channel Name"=w351, "Parent Ref in"=w371) -> ("error out"=w353:errorcluster)  [unwired: 2 in, 3 out]
                    }
                  }
                  n187 = call <vilib>:"NI VeriStand - Add Custom Device Section.vi"("error in (no error)"=w327, "Section Name"="Status Variables", "Parent Ref in"=w316) -> ("error out"=w323:errorcluster, "Section Ptr"=w321:T5)  [unwired: 5 in, 2 out]
                  n188 = call "Host - Lookup Remote IO ID.vi"() -> ("RemIO Module Out"=w319:refnum<class "RemIO Module.lvclass">)  [unwired: 10 in, 1 out]
                  n189 = call "Write RemIO Module Page Property.vi"("error in (no error)"=w323, "Node Ptr In"=w321, "RemIO Module"=w319) -> ("error out"=w322:errorcluster, "Node Ptr Out"=w320:T14)  [unwired: 6 in, 1 out]
                  n190 = for {
                    tunnel: w324 -> [w398] mode=indexing
                    tunnel: w320 -> [w399]
                    tunnel: [w378] -> w325
                    tunnel: w322 -> [w376]
                    w385 = refnum<k21> refnum  # I/O Variable
                    w395 = T12 {"Type"=enum."Input", "Units"="", "Default Value"=0.0, "Faultable"=FALSE, "Scalable"=FALSE}  # Channel
                    # "Creating a VS channel for each Status Variable"
                    # "Getting I/O VAR Data Type"
                    n191 = To More Specific Class(target class=w385, reference=w398, error in=w376) -> (specific class reference=w386:refnum<k21>, error out=w387:errorcluster)
                    n192 = property class="I/O Variable"(reference=w386, error in=w387) -> (error out=w397:errorcluster, "Name"=w396:string, "Writable"=w394:bool, "DataType"=w389:variant)  [unwired: 1 out]
                    n193 = case shown="True" w394 {
                      tunnel: [Custom_Device_Channel_Type."Output" ("Type") Custom_Device_Channel_Type."Input" ("Type")] -> w377
                      tunnel: [TRUE TRUE] -> w393
                      frame False {
                      }
                      frame True {
                      }
                    }
                    n194 = Variant To Flattened String(Variant=w389) -> (1:w390:i16[])  [unwired: 1 out]
                    n195 = Index Array(array=w390, index=1) -> (element=w392:i16)
                    n196 = call "TypeCodeToEnum.vi"("Type Code (numbers in hexadecimal)"=w392) -> (2:"UDV Data Type"=w388:string, 3:"UDV Data Type"=w380:T13)  [unwired: 9 in]
                    n197 = global read "Property Strings.vi" "Data Type"() -> (w383:string)
                    n198 = Bundle By Name(cluster=w395, "Type"=w377, "Units"=w388, "Faultable"=w393, "Scalable"=w393) -> (w384:T12)
                    n199 = To Long Integer(number=w380) -> (32bit integer=w381:i32)
                    n200 = Build Array(w381) -> (w379:i32[])
                    n201 = Build Array(w383) -> (w382:string[])
                    n202 = call <vilib>:"NI VeriStand - Add Custom Device Channel.vi"("Property Values"=w379, "Property names"=w382, "error in (no error)"=w397, "Channel"=w384, "Channel Name"=w396, "Parent Ref in"=w399) -> ("error out"=w378:errorcluster)  [unwired: 2 in, 3 out]
                  }
                }
              }
            }
          }
          n203 = Unbundle By Name(w18) -> ("Local Chassis.Modules"=w17:T9[])
          n204 = Empty Array?(array=w17) -> (empty?=w16:bool)
          n205 = case shown="False" w16 {
            tunnel: w20 -> [w453 w511]
            tunnel: w19 -> [w452 _]
            tunnel: w17 -> [w451 _]
            tunnel: [w422 w511] -> w15
            frame False {
              # "Add code to handle case where\nbitfile is found?"
              n206 = global read "Property Strings.vi" "# Slots"() -> (w449:string)
              n207 = global read "Scan Engine GUIDs.vi" "Local Chassis"() -> (w450:string)
              n208 = Build Array(8 ("# Slots")) -> (w447:i32[])
              n209 = Build Array(w449) -> (w448:string[])
              n210 = call <vilib>:"NI VeriStand - Add Custom Device Section.vi"("Property Values"=w447, "Property names"=w448, "GUID (Default Section)"=w450, "error in (no error)"=w453, "Section Name"="Local Chassis", "Parent Ref in"=w452) -> ("error out"=w444:errorcluster, "Section Ptr"=w442:T5)  [unwired: 2 in, 2 out]
              n211 = for {
                N: 8 -> [_]
                shift-right: [w455] -> w446
                shift-left: w444 -> [w461]
                shift-right: [w478] -> w445
                shift-left: w442 -> [w483]
                tunnel: w451 -> [w466]
                i -> [w480]
                n212 = Increment(x=w480) -> (x+1=w465:i32)
                n213 = for {
                  tunnel: w466 -> [w510] mode=indexing
                  tunnel: w465 -> [w508]
                  tunnel: [w507] -> w464
                  tunnel: [w506] -> w459
                  stop <- w507 stop-if-true
                  (unwired) u32 0 ("Model")
                  n214 = Unbundle By Name(w510) -> ("Model"=w506:u32, "Slot"=w509:u32)
                  n215 = Equal?(x=w509, y=w508) -> (x = y?=w507:bool)
                }
                n216 = case shown="False" w464 {
                  tunnel: [" (Empty)" ("Section Name") w489] -> w463
                  tunnel: [Module_Models."Empty" ("Module") w496] -> w462
                  tunnel: w461 -> [w485 w497]
                  tunnel: [w485 w498] -> w460
                  tunnel: w459 -> [_ w495]
                  tunnel: [w484 w488] -> w454
                  frame False {
                    n217 = global read "Scan Engine GUIDs.vi" "Slot - Empty"() -> (w484:string)
                  }
                  frame True {
                    n218 = Number To Decimal String(number=w495) -> (decimal integer string=w494:string)  [unwired: 1 in]
                    n219 = Concatenate Strings("NI " ("string"), w494) -> (w492:string)
                    n220 = Concatenate Strings(" (" ("string"), w492, ")" ("string")) -> (w489:string)
                    n221 = Scan From String(format string="%s", input string=w492, error in=w497, default 1=Module_Models."Empty" ("Module")) -> (error out=w499:errorcluster, output 1=w496:T3)  [unwired: 1 in, 2 out]
                    n222 = Unbundle By Name(w499) -> ("code"=w500:i32)
                    n223 = case shown="0, Default" w500 {
                      tunnel: [w503 w504] -> w498
                      tunnel: w499 -> [w503 w505]
                      frame 0, Default {
                      }
                      frame 85 {
                        n224 = call <vilib>:"Clear Errors.vi"("error in (no error)"=w505) -> ("error out"=w504:errorcluster)  [unwired: 5 in, 1 out]
                      }
                    }
                    n225 = global read "Scan Engine GUIDs.vi" "Slot"() -> (w488:string)
                  }
                }
                n226 = Bundle By Name(cluster=T2 {"Slot"=0, "EtherCAT?"=FALSE} ("Slot Settings"), "Slot"=w465, "EtherCAT?"=FALSE) -> (w475:T2)
                n227 = Number To Decimal String(number=w465, width (-)=i16 1) -> (decimal integer string=w482:string)
                n228 = call "Init Module.vi"("error in (no error)"=w460, "Slot Settings"=w475, "Module Model"=w462) -> ("error out"=w470:errorcluster, "RSI Module out"=w456:refnum<class "RSI Module.lvclass">)  [unwired: 7 in]
                n229 = global read "Class Property Strings.vi" "Module Class"() -> (w468:string)
                n230 = Concatenate Strings("Slot" ("string"), w482, w463) -> (w479:string)
                n231 = Flatten To String(anything=w456, error in (no error)=w470) -> (data string=w471:string, error out=w469:errorcluster)  [unwired: 2 in, 1 out]
                n232 = To Variant(anything=w471) -> (Variant=w476:variant)
                n233 = Build Array(w476) -> (w477:variant[])
                n234 = Build Array(w468) -> (w472:string[])
                n235 = call <vilib>:"NI VeriStand - Add Custom Device Section.vi"("Property Values"=w477, "Property names"=w472, "GUID (Default Section)"=w454, "error in (no error)"=w469, "Section Name"=w479, "Parent Ref in"=w483) -> ("error out"=w457:errorcluster, "Section Ptr"=w458:T5, "Parent Ref out"=w478:T5)  [unwired: 2 in, 1 out]
                n236 = call-dynamic "Create Channels.vi"("error in (no error)"=w457, "RSI Module in"=w456, "Parent Ref in"=w458) -> ("error out"=w455:errorcluster)  [unwired: 6 in, 2 out]
              }
              n237 = global read "Property Strings.vi" "Bitfile Path - Target"() -> (w436:string)
              n238 = global read "Property Strings.vi" "Bitfile Path - Host"() -> (w433:string)
              n239 = global read "Property Strings.vi" "FPGA Target"() -> (w434:string)
              n240 = global read "Property Strings.vi" "FPGA Sig"() -> (w435:string)
              n241 = To Variant(anything=path "") -> (Variant=w437:variant)
              n242 = To Variant(anything="") -> (Variant=w439:variant)
              n243 = Build Array(w433, w434, w435, w436) -> (w431:string[])
              n244 = Build Array(w437, w439, w439, w437) -> (w430:variant[])
              n245 = global read "Scan Engine GUIDs.vi" "User Vars Page - Local"() -> (w429:string)
              n246 = call <vilib>:"NI VeriStand - Add Custom Device Section.vi"("Property Values"=w430, "Property names"=w431, "GUID (Default Section)"=w429, "error in (no error)"=w446, "Section Name"="User Variables", "Parent Ref in"=w445) -> ("error out"=w425:errorcluster, "Section Ptr"=w426:T5)  [unwired: 2 in, 2 out]
              n247 = global read "String Constants.vi" "Local FPGA Desc"() -> (w428:string)
              n248 = call <vilib>:"NI VeriStand - Set Item Description.vi"("error in (no error)"=w425, "Description"=w428, "Item Ref in"=w426) -> ("error out"=w423:errorcluster, "Item Ref out"=w421:T5)  [unwired: 6 in, 1 out]
              n249 = call "Set FPGA Mode.vi"("error in (no error)"=w423, "FPGAScanInterfaceMode"=Host_-_FPGAScanInterfaceMode."Scan Mode", "Item Ref in"=w421) -> ("error out"=w422:errorcluster)  [unwired: 7 in, 1 out]
            }
            frame True {
            }
          }
          n250 = flat-sequence {
            tunnel: w15 -> [w35]
            tunnel: [w33] -> w14
            frame #0 {
              n251 = call <vilib>:"NI VeriStand - Commit System Explorer Update Buffer.vi"() -> ("error out"=w34:errorcluster)  [unwired: 11 in]
              n252 = Merge Errors(w35, w34) -> (w33:errorcluster)
            }
          }
        }
      }
    }
    frame Error {
    }
  }
  n253 = call <vilib>:"Simple Error Handler.vi"("error in (no error)"=w2) -> ("error out"=→"error out":errorcluster)  [unwired: 4 in, 4 out]
